vi "JKI SM Editor - Post-Build Custom Action.vi"(10 "Variant":variant) -> (0 "error out":errorcluster)   [LabVIEW 2020]
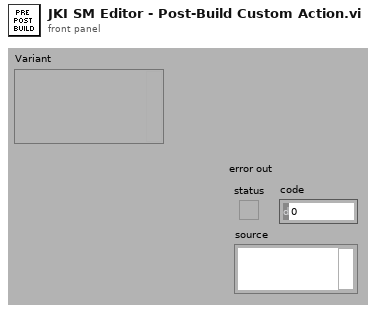
[diagram p1: front panel]
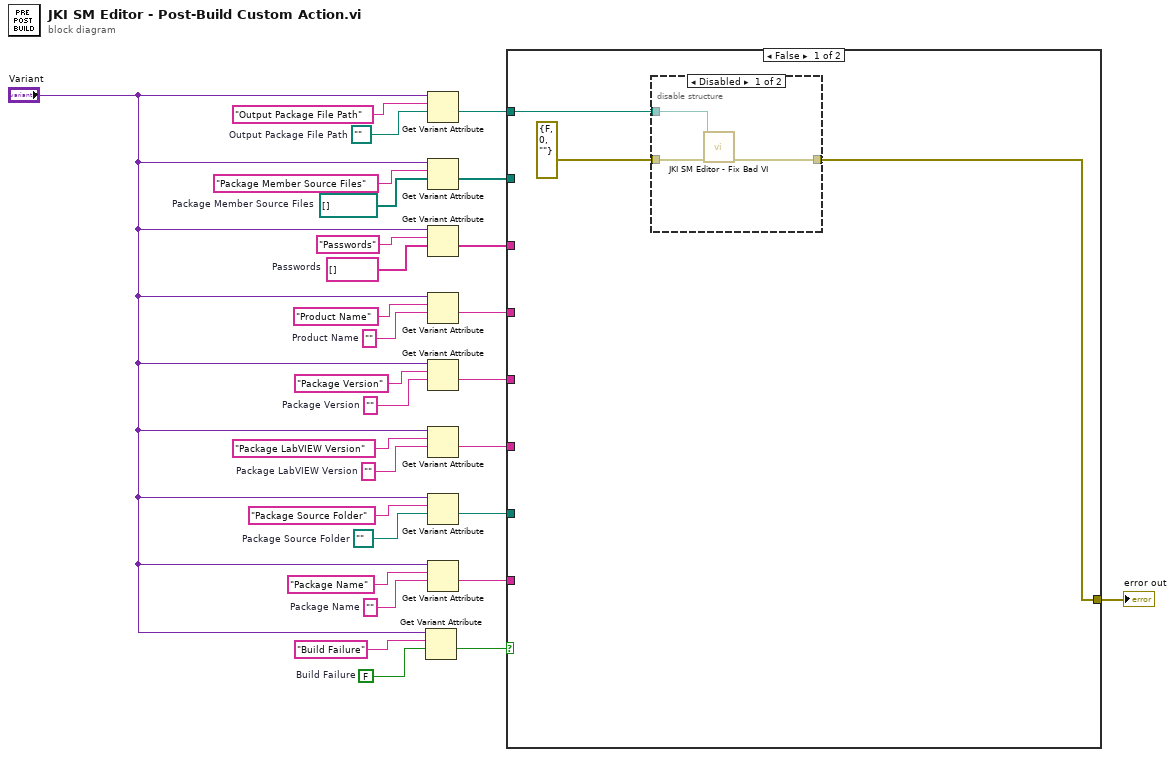
[diagram p0: block diagram]
diagram:
  w4 = FALSE  # Build Failure
  w14 = path ""  # Package Source Folder
  w15 = ""  # Package Name
  w18 = ""  # Package LabVIEW Version
  w20 = ""  # Package Version
  w22 = ""  # Product Name
  w24 = string[] []  # Passwords
  w26 = path[] []  # Package Member Source Files
  w28 = path ""  # Output Package File Path
  n1 = Get Variant Attribute(Variant="Variant", name="Build Failure", default value (empty Variant)=w4) -> (value=w1:bool)  [unwired: 1 in, 3 out]
  n2 = Get Variant Attribute(Variant="Variant", name="Output Package File Path", default value (empty Variant)=w28) -> (value=w13:path)  [unwired: 1 in, 3 out]
  n3 = Get Variant Attribute(Variant="Variant", name="Package Member Source Files", default value (empty Variant)=w26) -> (value=w12:path[])  [unwired: 1 in, 3 out]
  n4 = Get Variant Attribute(Variant="Variant", name="Passwords", default value (empty Variant)=w24) -> (value=w11:string[])  [unwired: 1 in, 3 out]
  n5 = Get Variant Attribute(Variant="Variant", name="Product Name", default value (empty Variant)=w22) -> (value=w10:string)  [unwired: 1 in, 3 out]
  n6 = Get Variant Attribute(Variant="Variant", name="Package Version", default value (empty Variant)=w20) -> (value=w9:string)  [unwired: 1 in, 3 out]
  n7 = Get Variant Attribute(Variant="Variant", name="Package LabVIEW Version", default value (empty Variant)=w18) -> (value=w8:string)  [unwired: 1 in, 3 out]
  n8 = Get Variant Attribute(Variant="Variant", name="Package Source Folder", default value (empty Variant)=w14) -> (value=w7:path)  [unwired: 1 in, 3 out]
  n9 = Get Variant Attribute(Variant="Variant", name="Package Name", default value (empty Variant)=w15) -> (value=w6:string)  [unwired: 1 in, 3 out]
  n10 = case shown="False" w1 {
    tunnel: w13 -> [w32 _]
    tunnel: w12 -> [_ _]
    tunnel: w11 -> [_ _]
    tunnel: w10 -> [_ _]
    tunnel: w9 -> [_ _]
    tunnel: w8 -> [_ _]
    tunnel: w7 -> [_ _]
    tunnel: w6 -> [_ _]
    tunnel: [w31 _] -> w2
    frame False {
      n11 = disable-structure shown="Disabled" {
        disable-tunnel: w32 -> [w35 _]
        disable-tunnel: [w34 w36] -> w31
        disable-tunnel: errorcluster {"status"=FALSE, "code"=0, "source"=""} ("error in (no error)") -> [w33 w36]
        frame Disabled {
          n12 = call "JKI SM Editor - Fix Bad VI.vi"("error in (no error)"=w33, "Output Package File Path"=w35) -> ("error out"=w34:errorcluster)  [unwired: 9 in]
        }
        frame Enabled {
        }
      }
    }
    frame True {
    }
  }
  "error out" <- w2
